vi "Input_Sensors_Conveyor_2.vi"() -> (3 "ConveyorV2 Inputs":T1={"Grab Ball Detector Count"=539, "Bottom Ball Detector Count"=541, "Top In Place Ball Detector Count"=3406, "Top Too Far Ball Detector Count"=0, "Top Not Far Enough"=0})   [LabVIEW 2012]
uses:
  Sensor_Input_ConveyorV2.ctl
panel:
  in  "Top not far enough max":dbl=11.0
  in  "Top not far enough min":dbl
  in  "Top too far distance min":dbl
  in  "Top too far distance max":dbl=11.0
  in  "Top in place distance min":dbl
  in  "Top in place distance max":dbl=6.0
  in  "Grab Distance Min":dbl
  in  "Grab Distance Max":dbl=8.0
  in  "Bottom Distance Max":dbl=6.0
  out "error out":errorcluster
  in  "Bottom Distance Min":dbl
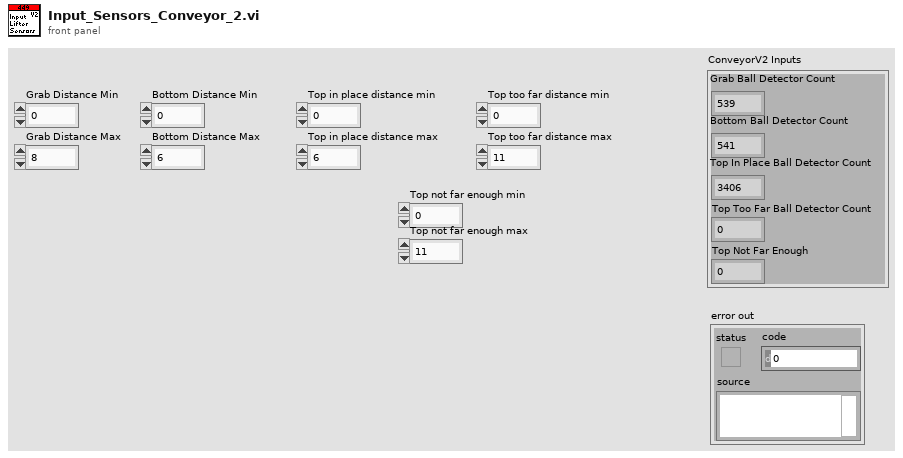
[diagram p1: front panel]
types:
  T1 = typedef "Sensor_Input_ConveyorV2.ctl" = cluster{"Grab Ball Detector Count":i32, "Bottom Ball Detector Count":i32, "Top In Place Ball Detector Count":i32, "Top Too Far Ball Detector Count":i32, "Top Not Far Enough":i32}
  T2 = typedef "WPI_AnalogChannelDevRef.ctl" = cluster{"DevStatus":errorcluster, "Analog Module":T3, "Analog Channel":T4}
  T3 = typedef "FPGA_TypedefAnalogModule.ctl" = enum16{"Analog Module 1", "Analog Module 2"}
  T4 = typedef "FPGA_AIChannel.ctl" = enum8{"AI 1", "AI 2", "AI 3", "AI 4", "AI 5", "AI 6", "AI 7", "AI 8", "Invalid"}
  T5 = typedef "WPI_DigitalInputDevRef.ctl" = cluster{"DevStatus":errorcluster, "DIO Channel":T6, "Digital Module":T7}
  T6 = typedef "FPGA_DIOChannel.ctl" = enum8{"DIO 1", "DIO 2", "DIO 3", "DIO 4", "DIO 5", "DIO 6", "DIO 7", "DIO 8", "DIO 9", "DIO 10", "DIO 11", "DIO 12", "DIO 13", "DIO 14", "Invalid"}
  T7 = typedef "FPGA_TypedefDigitalModule.ctl" = enum16{"Digital Module 1", "Digital Module 2"}
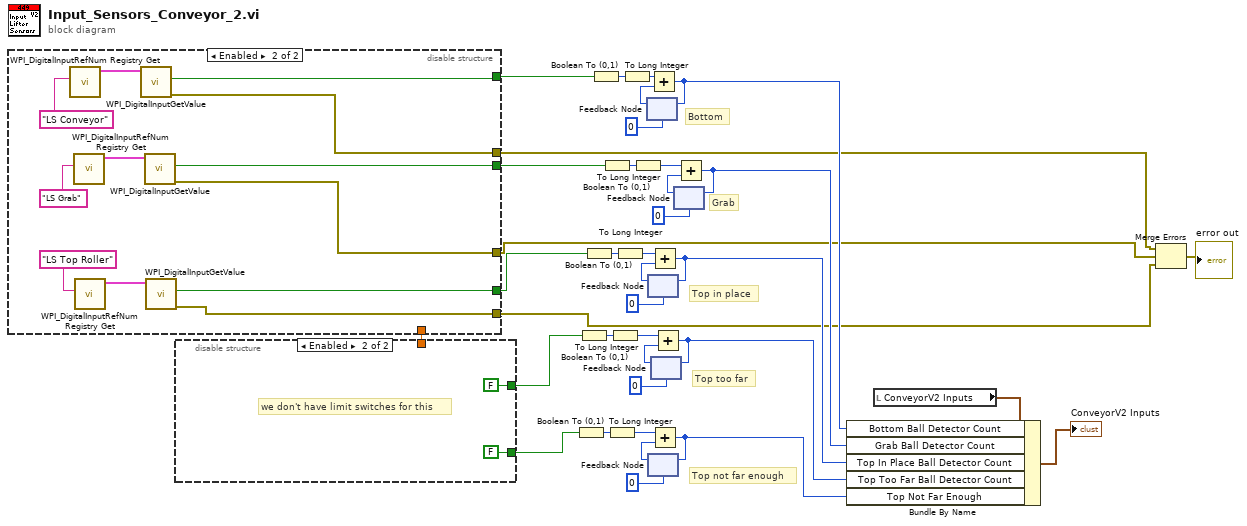
[diagram p0: block diagram]
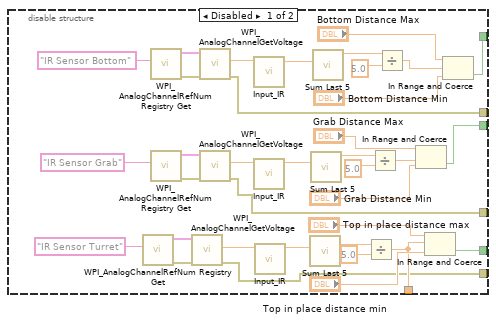
[diagram p2: hidden frame]
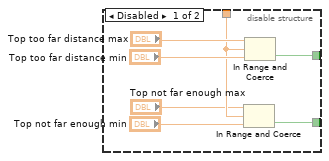
[diagram p3: hidden frame]
diagram:
  # "Top not far enough"
  # "Top too far"
  # "Top in place"
  # "Grab"
  # "Bottom"
  n1 = disable-structure shown="Enabled" {
    disable-tunnel: [w73 w75] -> w18
    disable-tunnel: [w72 w83] -> w17
    disable-tunnel: [w71 w79] -> w16
    disable-tunnel: [w59 _] -> w6
    disable-tunnel: [w40 w74] -> w3
    disable-tunnel: [w39 w82] -> w2
    disable-tunnel: [w38 w78] -> w1
    frame Disabled {
      n2 = call <vilib>:"WPI_AnalogChannelRefNum Registry Get.vi"("refnum name"="IR Sensor Turret" ("Reference Name")) -> ("error out"=w43:errorcluster, "AIDeviceRef"=w44:T2)  [unwired: 9 in]
      n3 = call <vilib>:"WPI_AnalogChannelRefNum Registry Get.vi"("refnum name"="IR Sensor Bottom" ("Reference Name")) -> ("error out"=w52:errorcluster, "AIDeviceRef"=w51:T2)  [unwired: 9 in]
      n4 = call <vilib>:"WPI_AnalogChannelRefNum Registry Get.vi"("refnum name"="IR Sensor Grab" ("Reference Name")) -> ("error out"=w48:errorcluster, "AIDeviceRef"=w47:T2)  [unwired: 9 in]
      n5 = call <vilib>:"WPI_AnalogChannelGetVoltage.vi"("error in (no error)"=w43, "AIDeviceRef"=w44) -> ("error out"=w38:errorcluster, "Voltage"=w42:dbl)  [unwired: 7 in, 1 out]
      n6 = call <vilib>:"WPI_AnalogChannelGetVoltage.vi"("error in (no error)"=w52, "AIDeviceRef"=w51) -> ("error out"=w40:errorcluster, "Voltage"=w50:dbl)  [unwired: 7 in, 1 out]
      n7 = call <vilib>:"WPI_AnalogChannelGetVoltage.vi"("error in (no error)"=w48, "AIDeviceRef"=w47) -> ("error out"=w39:errorcluster, "Voltage"=w46:dbl)  [unwired: 7 in, 1 out]
      n8 = call "Input_IR.vi"("Analog Input"=w50) -> ("Distance (in)"=w60:dbl)  [unwired: 10 in]
      n9 = call "Input_IR.vi"("Analog Input"=w46) -> ("Distance (in)"=w56:dbl)  [unwired: 10 in]
      n10 = call "Input_IR.vi"("Analog Input"=w42) -> ("Distance (in)"=w67:dbl)  [unwired: 10 in]
      n11 = call "Sum Last 5.vi"("Input"=w67) -> ("Sum Last 5"=w66:dbl)  [unwired: 10 in]
      n12 = call "Sum Last 5.vi"("Input"=w56) -> ("Sum Last 5"=w54:dbl)  [unwired: 10 in]
      n13 = call "Sum Last 5.vi"("Input"=w60) -> ("Sum Last 5"=w63:dbl)  [unwired: 10 in]
      n14 = Divide(x=w66, y=5.0) -> (x/y=w59:dbl)
      n15 = Divide(x=w54, y=5.0) -> (x/y=w55:dbl)
      n16 = Divide(x=w63, y=5.0) -> (x/y=w61:dbl)
      n17 = In Range and Coerce(upper limit="Grab Distance Max", x=w55, lower limit="Grab Distance Min") -> (In Range?=w72:bool)  [unwired: 1 out]
      n18 = In Range and Coerce(upper limit="Top in place distance max", x=w59, lower limit="Top in place distance min") -> (In Range?=w71:bool)  [unwired: 1 out]
      n19 = In Range and Coerce(upper limit="Bottom Distance Max", x=w61, lower limit="Bottom Distance Min") -> (In Range?=w73:bool)  [unwired: 1 out]
    }
    frame Enabled {
      n20 = call <vilib>:"WPI_DigitalInputRefNum Registry Get.vi"("refnum name"="LS Conveyor") -> ("DigitalInputDevRef"=w77:T5)  [unwired: 9 in, 1 out]
      n21 = call <vilib>:"WPI_DigitalInputRefNum Registry Get.vi"("refnum name"="LS Grab") -> ("DigitalInputDevRef"=w85:T5)  [unwired: 9 in, 1 out]
      n22 = call <vilib>:"WPI_DigitalInputRefNum Registry Get.vi"("refnum name"="LS Top Roller") -> ("DigitalInputDevRef"=w81:T5)  [unwired: 9 in, 1 out]
      n23 = call <vilib>:"WPI_DigitalInputGetValue.vi"("DigitalInputDevRef"=w77) -> ("error out"=w74:errorcluster, "Value"=w75:bool)  [unwired: 8 in, 1 out]
      n24 = call <vilib>:"WPI_DigitalInputGetValue.vi"("DigitalInputDevRef"=w85) -> ("error out"=w82:errorcluster, "Value"=w83:bool)  [unwired: 8 in, 1 out]
      n25 = call <vilib>:"WPI_DigitalInputGetValue.vi"("DigitalInputDevRef"=w81) -> ("error out"=w78:errorcluster, "Value"=w79:bool)  [unwired: 8 in, 1 out]
    }
  }
  n26 = disable-structure shown="Enabled" {
    disable-tunnel: [w90 FALSE] -> w15
    disable-tunnel: w6 -> [w89 _]
    disable-tunnel: [w86 FALSE] -> w5
    frame Disabled {
      n27 = In Range and Coerce(upper limit="Top not far enough max", x=w89, lower limit="Top not far enough min") -> (In Range?=w86:bool)  [unwired: 1 out]
      n28 = In Range and Coerce(upper limit="Top too far distance max", x=w89, lower limit="Top too far distance min") -> (In Range?=w90:bool)  [unwired: 1 out]
    }
    frame Enabled {
      # "we don't have limit switches for this"
    }
  }
  n29 = Boolean To (0,1)(Boolean=w5) -> (0, 1=w10:i16)
  n30 = Boolean To (0,1)(Boolean=w15) -> (0, 1=w26:i16)
  n31 = Boolean To (0,1)(Boolean=w16) -> (0, 1=w33:i16)
  n32 = Boolean To (0,1)(Boolean=w18) -> (0, 1=w37:i16)
  n33 = Boolean To (0,1)(Boolean=w17) -> (0, 1=w21:i16)
  n34 = To Long Integer(number=w10) -> (32bit integer=w7:i32)
  n35 = To Long Integer(number=w26) -> (32bit integer=w29:i32)
  n36 = To Long Integer(number=w33) -> (32bit integer=w30:i32)
  n37 = To Long Integer(number=w37) -> (32bit integer=w34:i32)
  n38 = To Long Integer(number=w21) -> (32bit integer=w24:i32)
  n39 = feedback #1(0) -> (w36:i32)
  n40 = feedback #2(0) -> (w32:i32)
  n41 = feedback #3(0) -> (w9:i32)
  n42 = Add(x=w34, y=w36) -> (x+y=w14:i32)
  n43 = feedback-in #1(w14) -> ()
  n44 = Add(x=w30, y=w32) -> (x+y=w12:i32)
  n45 = feedback-in #2(w12) -> ()
  n46 = Add(x=w7, y=w9) -> (x+y=w4:i32)
  n47 = feedback-in #3(w4) -> ()
  n48 = feedback #4(0) -> (w27:i32)
  n49 = Add(x=w29, y=w27) -> (x+y=w11:i32)
  n50 = feedback-in #4(w11) -> ()
  n51 = feedback #5(0) -> (w22:i32)
  n52 = Add(x=w24, y=w22) -> (x+y=w13:i32)
  n53 = feedback-in #5(w13) -> ()
  n54 = local read "ConveyorV2 Inputs"() -> (w19:T1)
  n55 = Bundle By Name(cluster=w19, "Bottom Ball Detector Count"=w14, "Grab Ball Detector Count"=w13, "Top In Place Ball Detector Count"=w12, "Top Too Far Ball Detector Count"=w11, "Top Not Far Enough"=w4) -> (→"ConveyorV2 Inputs":T1)
  n56 = Merge Errors(w3, w2, w1) -> (→"error out":errorcluster)
